vi "Create Plot Object.vi"(6 "Control Ref Queue":T1, 7 "Actual Transform In":T2, 8 "error in (no error)":errorcluster, 9 "Multiplot Representation In":T4, 10 "3D Surface.lvclass in":refnum<class "3D Surface.lvclass">, 11 "Plot Object In":refnum<vi>) -> (0 "error out":errorcluster, 1 "Multiplot Representation Out":T4, 2 "3D Surface.lvclass out":refnum<class "3D Surface.lvclass">, 3 "Plot Object Out":refnum<vi>, 5 "Actual Transform Out":T2)   [LabVIEW 2020, in "3D Surface.lvclass"]
uses:
  <vilib>/Math Plots/3D Math Plots/3D Surface/3D Surface/3D Surface.lvclass
  <vilib>/Math Plots/3D Math Plots/3D Plot/3D Plot/Typedef/Multiplot Representation.ctl
  <vilib>/Math Plots/3D Math Plots/3D Plot/3D Plot/Typedef/Plot Representation.ctl
  <vilib>/Math Plots/3D Math Plots/3D Plot/3D Plot/Typedef/Range Clusters.ctl
  <vilib>/Math Plots/3D Math Plots/3D Plot/3D Plot/Typedef/Mesh Data.ctl
  <vilib>/Math Plots/3D Math Plots/3D Plot/3D Plot/Typedef/Actual Transform.ctl
  <vilib>/Math Plots/3D Math Plots/3D Plot/Action String/3DMathPlot Ctrl Act Queue.ctl
  <vilib>/Math Plots/3D Math Plots/3D Plot/Action String/3DMathPlot Ctrl Act Cluster.ctl
  <vilib>/Math Plots/3D Math Plots/3D Plot/Action String/3DMathPlot State Class.ctl
  <vilib>/Math Plots/3D Math Plots/3D Surface/3D Surface/3D Surface.lvclass/3D Surface.ctl
  <vilib>/Math Plots/3D Math Plots/3D Plot/3D Plot/3D Plot.lvclass
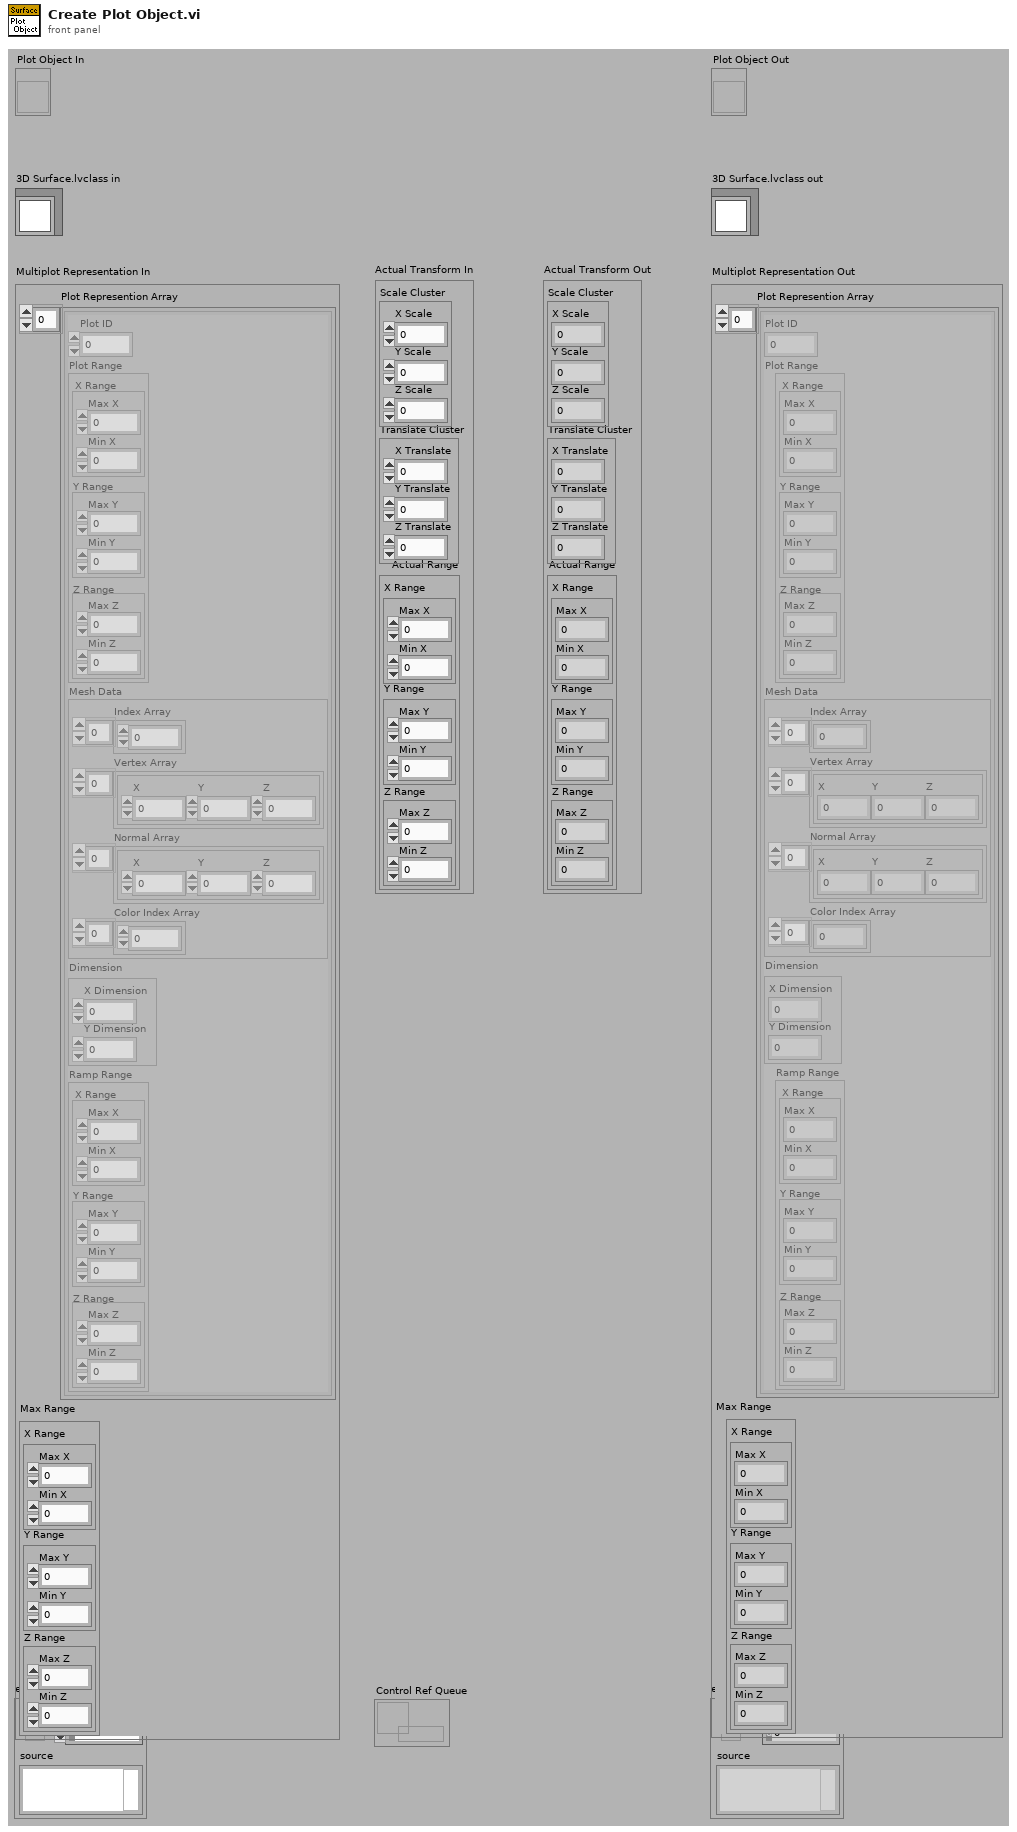
[diagram p1: front panel]
types:
  T1 = typedef "3DMathPlot Ctrl Act Queue.ctl" = refnum<queue>
  T2 = typedef "3D Plot.lvclass/Actual Transform.ctl" = cluster{"Scale Cluster":cluster{"X Scale":sgl, "Y Scale":sgl, "Z Scale":sgl}, "Translate Cluster":cluster{"X Translate":sgl, "Y Translate":sgl, "Z Translate":sgl}, "Actual Range":T3}
  T3 = typedef "3D Plot.lvclass/Range Clusters.ctl" = cluster{"X Range":cluster{"Max X":sgl, "Min X":sgl}, "Y Range":cluster{"Max Y":sgl, "Min Y":sgl}, "Z Range":cluster{"Max Z":sgl, "Min Z":sgl}}
  T4 = typedef "3D Plot.lvclass/Multiplot Representation.ctl" = cluster{"Plot Represention Array":T5[], "Max Range":T3}
  T5 = typedef "3D Plot.lvclass/Plot Representation.ctl" = cluster{"Plot ID":i32, "Plot Range":T3, "Mesh Data":T6, "Dimension":cluster{"X Dimension":i32, "Y Dimension":i32}, "Ramp Range":T3}
  T6 = typedef "3D Plot.lvclass/Mesh Data.ctl" = cluster{"Index Array":u32[], "Vertex Array":cluster{"X":sgl, "Y":sgl, "Z":sgl}[], "Normal Array":cluster{"X":sgl, "Y":sgl, "Z":sgl}[], "Color Index Array":i32[]}
  T7 = typedef "3D Surface.lvclass/3D Surface Property Array.ctl" = T8[]
  T8 = typedef "3D Surface.lvclass/3D Surface Property.ctl" = cluster{"General Property":cluster{"Plot Name":string, "Coordinate System":enum16{"Cartesian", "Cylindrical", "Spherical"}, "Opacity":sgl}, "Projection Property":cluster{"Draw XY":bool, "Draw YZ":bool, "Draw XZ":bool}, "Plot Property":cluster{"Draw Surface":bool, "Draw Mesh":bool, "Draw Normal":bool, "Color Ramp Cluster":T9, "Line Style":T10, "Line Width":sgl, "Line Color":u32, "Antialiasing":bool}, "Surface Property":cluster{"Color Mode":enum16{"Flat Shading", "Interpolated Shading"}}}
  T9 = typedef "3D Plot.lvclass/Color Ramp Cluster.ctl" = cluster{"Color Ramp Style":enum16{"None", "Shaded", "Color spectrum", "Grey scale", "Custom"}, "Color Ramp Array":u32[], "Color Ramp Index":i32[], "Interpolate?":bool, "Logarithm?":bool}
  T10 = typedef "3D Plot.lvclass/Line Type.ctl" = enum16{"None", "Solid", "Dash", "Dot", "Dash Dot"}
  T11 = enum16{"Points", "Lines", "Line Strip", "Line Loop", "Triangles", "Triangle Strip", "Triangle Fan", "Quads", "Quad Strip", "Polygon"}
  T12 = cluster{"Draw XY":bool, "Draw YZ":bool, "Draw XZ":bool}
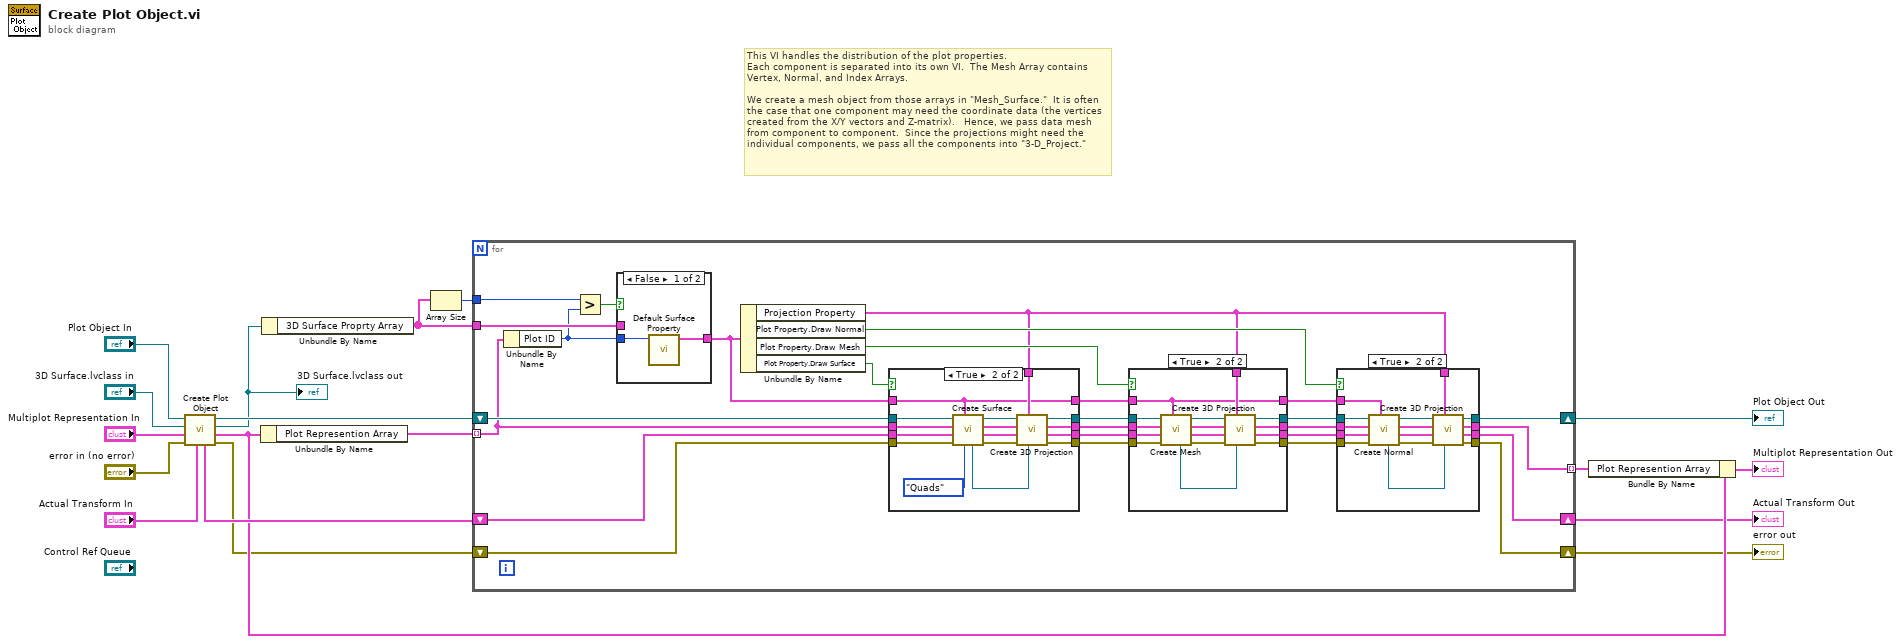
[diagram p0: block diagram]
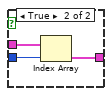
[diagram p2: hidden frame]
diagram:
  # "This VI handles the distribution of the plot properties.  \nEach component is separated into its own VI.  The Mesh Array contains Vertex, Normal, and Index Arrays.  \n\nWe create a mesh object from those arrays in \"Mesh_Surface.\"  It is often the case that one component may need the coordinate data (the vertices created from the X/Y vectors and Z-matrix).   Hence, we pass data mesh from component to component.  Since the projections might need the individual components, we pass all the components into \"3-D_Project.\""
  n1 = call-parent "Create Plot Object.vi"("Actual Transform In"="Actual Transform In", "error in (no error)"="error in (no error)", "Multiplot Representation In"="Multiplot Representation In", "3D Plot.lvclass in"="3D Surface.lvclass in", "Plot Object In"="Plot Object In") -> ("error out"=w7:errorcluster, "Multiplot Representation Out"=w11:T4, "3D Plot.lvclass out"=w3:refnum<class "3D Surface.lvclass">, "Plot Object Out"=w6:refnum<vi>, "Actual Transform Out"=w15:T2)  [unwired: 1 in, 1 out]
  "3D Surface.lvclass out" <- w3
  n2 = Unbundle By Name(w11) -> ("Plot Represention Array"=w4:T5[])
  n3 = Unbundle By Name(w3) -> ("3D Surface Proprty Array"=w2:T7)
  n4 = Array Size(array=w2) -> (size(s)=w1:i32)
  n5 = for {
    shift-right: [w31] -> w8
    shift-left: w7 -> [w41]
    shift-right: [w35] -> w5
    shift-left: w6 -> [w44]
    shift-right: [w32] -> w9
    shift-left: w15 -> [w42]
    tunnel: w4 -> [w43] mode=indexing
    tunnel: [w33] -> w18 mode=indexing
    tunnel: w2 -> [w45]
    tunnel: w1 -> [w20]
    n6 = Unbundle By Name(w43) -> ("Plot ID"=w21:i32)
    n7 = Greater?(x=w20, y=w21) -> (0:w19:bool)
    n8 = case shown="False" w19 {
      tunnel: w45 -> [_ w50]
      tunnel: [w47 w49] -> w36
      tunnel: w21 -> [w46 w48]
      frame False {
        n9 = call <vilib>:"Default Surface Property.vi"("Plot ID"=w46) -> ("Default Property"=w47:T8)  [unwired: 10 out]
      }
      frame True {
        n10 = Index Array(array=w50, index=w48) -> (element=w49:T8)
      }
    }
    n11 = Unbundle By Name(w36) -> ("Projection Property"=w24:T12, "Plot Property.Draw Normal"=w25:bool, "Plot Property.Draw Mesh"=w27:bool, "Plot Property.Draw Surface"=w26:bool)
    n12 = case shown="True" w26 {
      tunnel: w44 -> [w92 w107]
      tunnel: w43 -> [w91 w106]
      tunnel: w42 -> [w90 w105]
      tunnel: w41 -> [w89 w104]
      tunnel: [w89 w101] -> w40
      tunnel: [w90 w100] -> w39
      tunnel: [w91 w99] -> w38
      tunnel: [w92 w97] -> w37
      tunnel: w36 -> [w88 w93]
      tunnel: w24 -> [_ w94]
      tunnel: [w88 w93] -> w23
      frame False {
      }
      frame True {
        n13 = call <vilib>:"Create Surface.vi"("Draw Mode"=T11."Quads", "3D Surface Property"=w93, "error in (no error)"=w104, "Actual Transform In"=w105, "Plot Representation In"=w106, "Plot Object In"=w107) -> ("error out"=w103:errorcluster, "Actual Transform Out"=w102:T2, "Plot Representation Out"=w99:T5, "Plot Object Out"=w98:refnum<vi>, "Surface Object Out"=w96:refnum<vi>)  [unwired: 1 in]
        n14 = call <vilib>:"Create 3D Projection.vi"("Sub Object In"=w96, "Projection Property"=w94, "error in (no error)"=w103, "Actual Transform In"=w102, "Plot Object In"=w98) -> ("error out"=w101:errorcluster, "Actual Transform Out"=w100:T2, "Plot Object Out"=w97:refnum<vi>)  [unwired: 1 in, 3 out]
      }
    }
    n15 = case shown="True" w27 {
      tunnel: w40 -> [w70 w87]
      tunnel: w39 -> [w71 w86]
      tunnel: w38 -> [w72 w85]
      tunnel: w37 -> [w73 w84]
      tunnel: w23 -> [w69 w74]
      tunnel: w24 -> [_ w79]
      tunnel: [w73 w78] -> w34
      tunnel: [w70 w77] -> w30
      tunnel: [w71 w76] -> w29
      tunnel: [w72 w75] -> w28
      tunnel: [w69 w74] -> w22
      frame False {
      }
      frame True {
        n16 = call <vilib>:"Create Mesh.vi"("3D Surface Property"=w74, "error in (no error)"=w87, "Actual Transform In"=w86, "Plot Representation In"=w85, "Plot Object In"=w84) -> ("error out"=w83:errorcluster, "Actual Transform Out"=w81:T2, "Plot Representation Out"=w75:T5, "Plot Object Out"=w82:refnum<vi>, "Mesh Object Out"=w80:refnum<vi>)  [unwired: 1 in, 1 out]
        n17 = call <vilib>:"Create 3D Projection.vi"("Sub Object In"=w80, "Projection Property"=w79, "error in (no error)"=w83, "Actual Transform In"=w81, "Plot Object In"=w82) -> ("error out"=w77:errorcluster, "Actual Transform Out"=w76:T2, "Plot Object Out"=w78:refnum<vi>)  [unwired: 1 in, 3 out]
      }
    }
    n18 = case shown="True" w25 {
      tunnel: w22 -> [_ w68]
      tunnel: [w54 w65] -> w35
      tunnel: w24 -> [_ w64]
      tunnel: w34 -> [w54 w63]
      tunnel: [w53 w62] -> w33
      tunnel: [w52 w60] -> w32
      tunnel: [w51 w58] -> w31
      tunnel: w30 -> [w51 w57]
      tunnel: w29 -> [w52 w56]
      tunnel: w28 -> [w53 w55]
      frame False {
      }
      frame True {
        n19 = call <vilib>:"Create Normal.vi"("3D Surface Property"=w68, "error in (no error)"=w57, "Actual Transform In"=w56, "Plot Representation In"=w55, "Plot Object In"=w63) -> ("error out"=w59:errorcluster, "Actual Transform Out"=w61:T2, "Plot Representation Out"=w62:T5, "Plot Object Out"=w66:refnum<vi>, "Normal Object Out"=w67:refnum<vi>)  [unwired: 2 out]
        n20 = call <vilib>:"Create 3D Projection.vi"("Sub Object In"=w67, "Projection Property"=w64, "error in (no error)"=w59, "Actual Transform In"=w61, "Plot Object In"=w66) -> ("error out"=w58:errorcluster, "Actual Transform Out"=w60:T2, "Plot Object Out"=w65:refnum<vi>)  [unwired: 1 in, 3 out]
      }
    }
  }
  "error out" <- w8
  "Plot Object Out" <- w5
  "Actual Transform Out" <- w9
  n21 = Bundle By Name(cluster=w11, "Plot Represention Array"=w18) -> (→"Multiplot Representation Out":T4)
